vi "Helium Level Notification.vi"(0 "Recipient's Email Address":string="rongpu.zhou@levylab.org\n4125156650@txt.att.net", 1 "CC - Optional":string="4125156650@txt.att.net") -> ()   [LabVIEW 2013]
uses:
  PPMS Global.vi
panel:
  in  "Attachment - Optional":path
  # "Note: To send text message to AT&T cell phone, use email YOUR_NUMBER@txt.att.net"
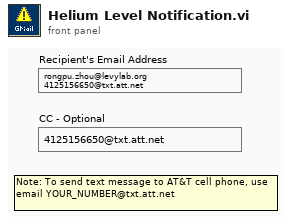
[diagram p1: front panel]
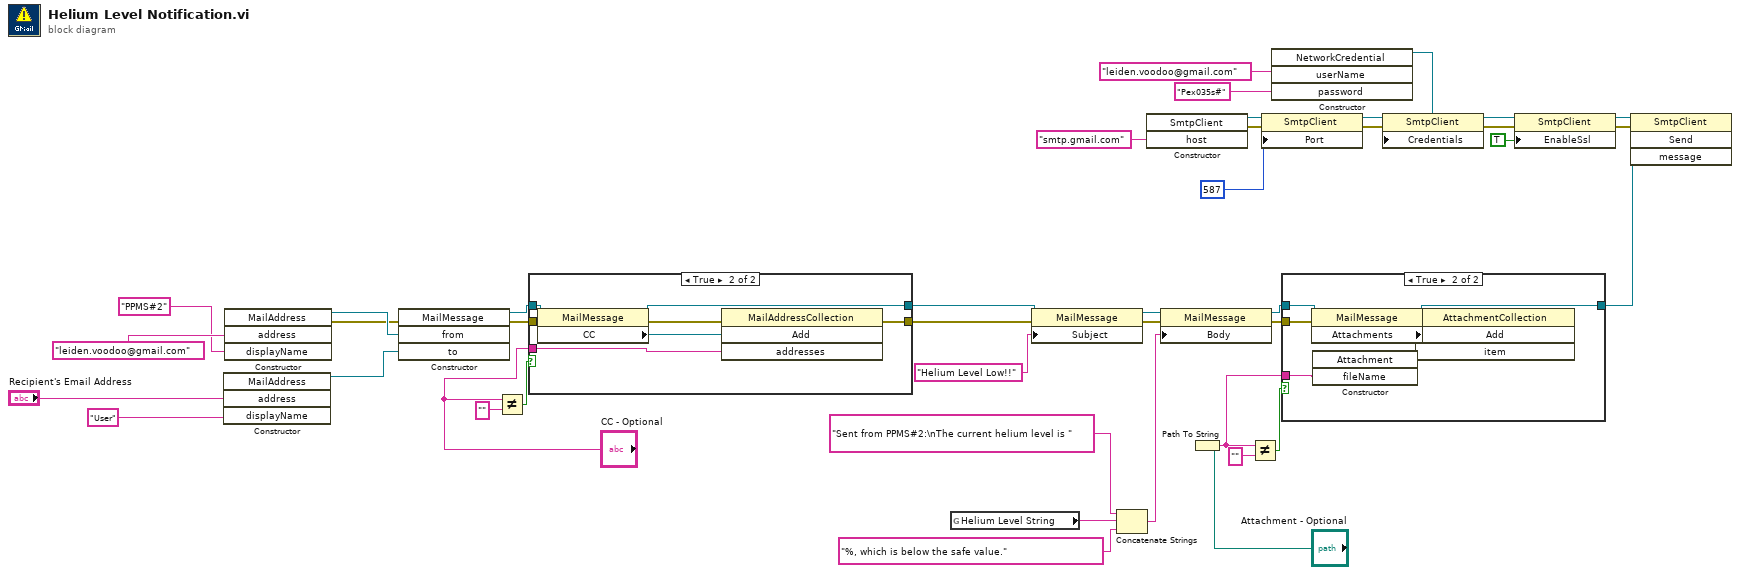
[diagram p0: block diagram]
diagram:
  n1 = constructor class="MailAddress"("address"="Recipient's Email Address", "displayName"="User" ("Recipient's Name")) -> (reference out=w42:refnum<k24>)  [unwired: 3 in, 4 out]
  n2 = constructor class="MailAddress"("address"="leiden.voodoo@gmail.com" ("Sender's Email Address (eg: LabVIEW@gmail.com)"), "displayName"="PPMS#2" ("Sender's Name")) -> (reference out=w41:refnum<k24>, error out=w6:errorcluster)  [unwired: 3 in, 3 out]
  n3 = constructor class="MailMessage"(error in=w6, "from"=w41, "to"=w42) -> (reference out=w13:refnum<k24>, error out=w12:errorcluster)  [unwired: 2 in, 3 out]
  n4 = Not Equal?(x="CC - Optional", y="") -> (x != y?=w15:bool)
  n5 = case shown="True" w15 {
    tunnel: "CC - Optional" -> [_ w49]
    tunnel: w13 -> [w44 w48]
    tunnel: w12 -> [w43 w47]
    tunnel: [w44 w46] -> w11
    tunnel: [w43 w45] -> w10
    frame False {
    }
    frame True {
      n6 = property class="MailMessage"(reference=w48, error in=w47) -> (reference out=w46:refnum<k24>, error out=w51:errorcluster, "CC"=w50:refnum<k24>)
      n7 = invoke class="MailAddressCollection" method="Add"(reference=w50, error in=w51, "addresses"=w49) -> (error out=w45:errorcluster)  [unwired: 1 in, 3 out]
    }
  }
  n8 = global read "PPMS Global.vi" "Helium Level String"() -> (w2:string)
  n9 = property class="MailMessage"(reference=w11, error in=w10, "Subject"="Helium Level Low!!") -> (reference out=w33:refnum<k24>, error out=w40:errorcluster)
  n10 = Concatenate Strings("Sent from PPMS#2:\nThe current helium level is " ("string"), w2, "%, which is below the safe value." ("string")) -> (w3:string)
  n11 = constructor class="SmtpClient"("host"="smtp.gmail.com" ("Outgoing Mail Server (SMTP)")) -> (reference out=w27:refnum<k24>, error out=w24:errorcluster)  [unwired: 3 in, 2 out]
  n12 = property class="MailMessage"(reference=w33, error in=w40, "Body"=w3) -> (reference out=w21:refnum<k24>, error out=w5:errorcluster)
  n13 = Path To String(path="Attachment - Optional") -> (string=w17:string)
  n14 = Not Equal?(x=w17, y="") -> (x != y?=w18:bool)
  n15 = property class="SmtpClient"(reference=w27, error in=w24, "Port"=587) -> (reference out=w26:refnum<k24>, error out=w23:errorcluster)
  n16 = constructor class="NetworkCredential"("userName"="leiden.voodoo@gmail.com" ("GMAIL Account User ID"), "password"="Pex035s#" ("GMAIL Account Password")) -> (reference out=w28:refnum<k24>)  [unwired: 3 in, 4 out]
  n17 = case shown="True" w18 {
    tunnel: w21 -> [w52 w56]
    tunnel: [w52 w55] -> w9
    tunnel: w17 -> [_ w54]
    tunnel: w5 -> [_ w53]
    frame False {
    }
    frame True {
      n18 = property class="MailMessage"(reference=w56, error in=w53) -> (reference out=w55:refnum<k24>, error out=w59:errorcluster, "Attachments"=w57:refnum<k24>)
      n19 = constructor class="Attachment"("fileName"=w54) -> (reference out=w58:refnum<k24>)  [unwired: 3 in, 3 out]
      n20 = invoke class="AttachmentCollection" method="Add"(reference=w57, error in=w59, "item"=w58) -> ()  [unwired: 1 in, 4 out]
    }
  }
  n21 = property class="SmtpClient"(reference=w26, error in=w23, "Credentials"=w28) -> (reference out=w25:refnum<k24>, error out=w22:errorcluster)
  n22 = property class="SmtpClient"(reference=w25, error in=w22, "EnableSsl"=TRUE ("Enable SSL")) -> (reference out=w7:refnum<k24>, error out=w8:errorcluster)
  n23 = invoke class="SmtpClient" method="Send"(reference=w7, error in=w8, "message"=w9) -> ()  [unwired: 1 in, 4 out]
